vi "read_tcx_file.vi"(8 "error in":errorcluster, 11 "File Path":path) -> (0 "error out":errorcluster, 2 "Time":timestamp[](array[timestamp]), 3 "Bmp":i32[](array[numeric]))   [LabVIEW 2025]
panel:
  out "error out 2":errorcluster
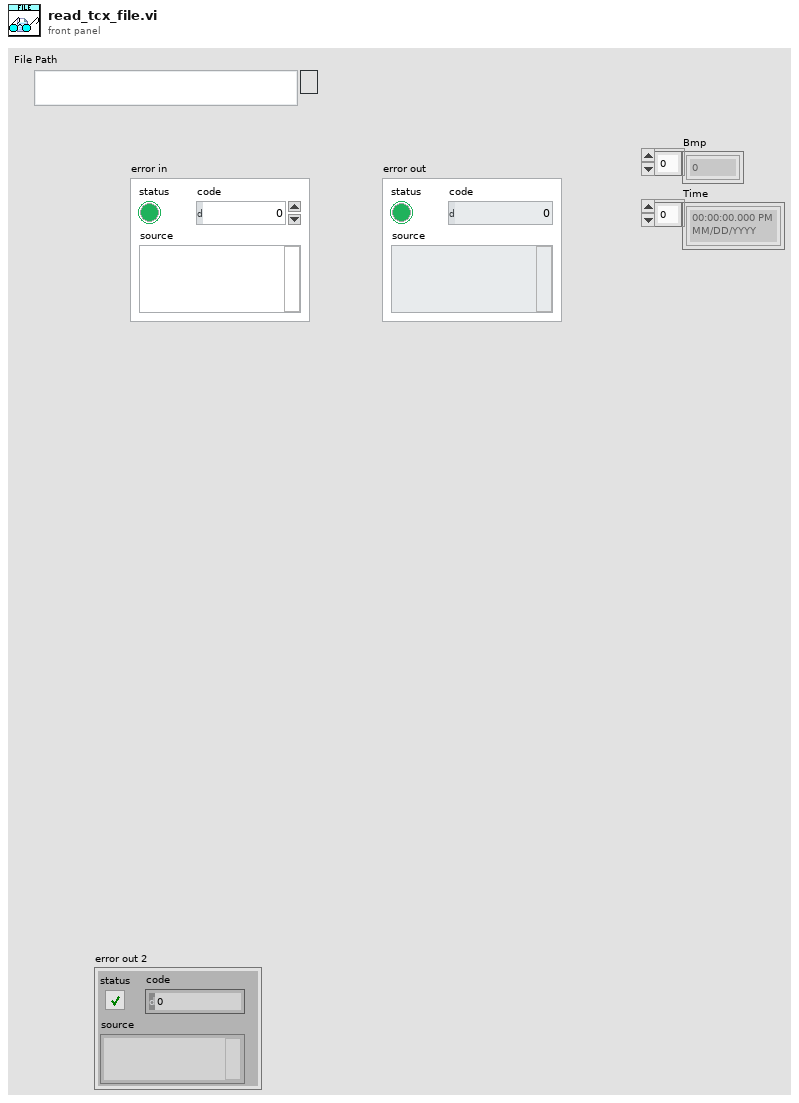
[diagram p1: front panel]
types:
  T1 = enum16{"open", "replace", "create", "open or create", "replace or create", "replace or create with confirmation"}
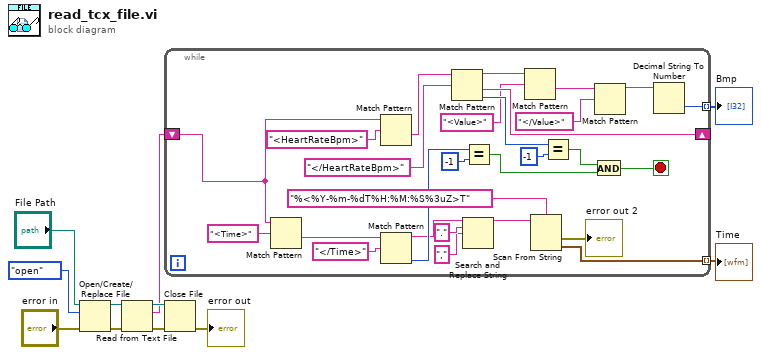
[diagram p0: block diagram]
diagram:
  n1 = Open/Create/Replace File(file path (use dialog)="File Path", error in="error in", operation (0:open)=T1."open") -> (refnum out=w5:refnum<file>, error out=w9:errorcluster)  [unwired: 3 in, 1 out]
  n2 = Read from Text File(file (use dialog)=w5, error in=w9) -> (refnum out=w4:refnum<file>, text=w3:string, error out=w8:errorcluster)  [unwired: 2 in, 1 out]
  n3 = while {
    shift-right: [w37] -> _
    shift-left: w3 -> [w27]
    tunnel: [w28] -> w2 mode=indexing
    tunnel: [w15] -> w1 mode=indexing
    stop <- w14 stop-if-true
    n4 = Match Pattern(string=w27, regular expression="<Time>") -> (after substring=w24:string)  [unwired: 1 in, 3 out]
    n5 = Match Pattern(string=w27, regular expression="<HeartRateBpm>") -> (after substring=w29:string)  [unwired: 1 in, 3 out]
    n6 = Match Pattern(string=w24, regular expression="</Time>") -> (before substring=w20:string, offset past match=w23:i32)  [unwired: 1 in, 2 out]
    n7 = Match Pattern(string=w29, regular expression="</HeartRateBpm>") -> (before substring=w30:string, after substring=w37:string, offset past match=w36:i32)  [unwired: 1 in, 1 out]
    n8 = Search and Replace String(input string=w20, search string=".", replace string="," ("replace string (\"\")")) -> (result string=w17:string)  [unwired: 5 in, 3 out]
    n9 = Equal?(x=w23, y=-1) -> (x = y?=w12:bool)
    n10 = Match Pattern(string=w30, regular expression="<Value>") -> (after substring=w33:string)  [unwired: 1 in, 3 out]
    n11 = Scan From String(format string="%<%Y-%m-%dT%H:%M:%S%3uZ>T", input string=w17) -> (error out=→"error out 2":errorcluster, output 1=w15:timestamp)  [unwired: 3 in, 2 out]
    n12 = Equal?(x=w36, y=-1) -> (x = y?=w13:bool)
    n13 = And(x=w13, y=w12) -> (x .and. y?=w14:bool)
    n14 = Match Pattern(string=w33, regular expression="</Value>") -> (before substring=w31:string)  [unwired: 1 in, 3 out]
    n15 = Decimal String To Number(string=w31) -> (number=w28:i32)  [unwired: 2 in, 1 out]
  }
  "Bmp" <- w2
  "Time" <- w1
  n16 = Close File(refnum=w4, error in=w8) -> (error out=→"error out":errorcluster)  [unwired: 1 out]
